vi "[FP] - VIG_Get Controls by Name.vi"(7 "MAin Ref\nFirst Time Only":refnum<vi>, 8 "Error":errorcluster, 11 "Control Names":string[](array[string])) -> (0 "Error Out":errorcluster, 3 "FP Controls Out":refnum<vi>[](array[refnum]), 5 "FrontPanel Out":refnum<vi>)   [LabVIEW 2015]
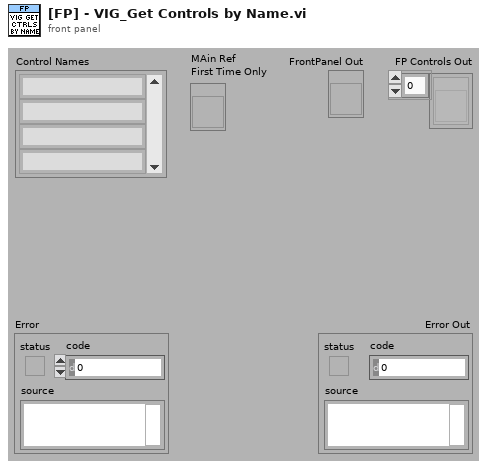
[diagram p1: front panel]
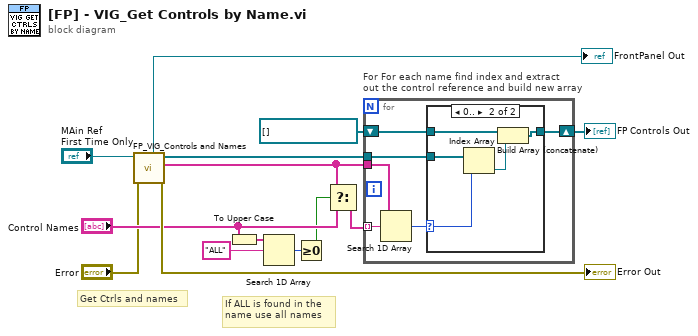
[diagram p0: block diagram]
diagram:
  # "If ALL is found in the\nname use all names"
  # "Get Ctrls and names"
  n1 = call "FP_VIG_Controls and Names.vi"("Error"="Error", "MAin Ref\nFirst Time only"="MAin Ref\nFirst Time Only") -> ("Error Out"=→"Error Out":errorcluster, "FP Names Out"=w8:string[], "FP Controls Out"=w3:refnum<vi>[], "FrontPanel Out"=→"FrontPanel Out":refnum<vi>)  [unwired: 6 in]
  n2 = To Upper Case(1:"Control Names") -> (0:w5:string[])
  n3 = Search 1D Array(1D array=w5, element="ALL") -> (index of element=w6:i32)  [unwired: 1 in]
  n4 = Greater Or Equal To 0?(x=w6) -> (x >= 0?=w7:bool)
  n5 = Select(t=w8, s=w7, f="Control Names") -> (s? t:f=w10:string[])
  n6 = for "For For each name find index and extract\nout the control reference and build new array" {
    tunnel: w8 -> [w20]
    tunnel: w10 -> [w19] mode=indexing
    tunnel: w3 -> [w17]
    shift-right: [w16] -> w14
    shift-left: refnum<vi>[] [] -> [w15]
    n7 = Search 1D Array(1D array=w20, element=w19) -> (index of element=w18:i32)  [unwired: 1 in]
    n8 = case shown="0.." w18 {
      selector: w18 -> [_ w25]
      tunnel: w17 -> [_ w26]
      tunnel: [w21 w23] -> w16
      tunnel: w15 -> [w21 w22]
      frame ..-1 {
      }
      frame 0.. {
        n9 = Index Array(array=w26, index=w25) -> (element=w24:refnum<vi>)
        n10 = Build Array (concatenate)(w22, w24) -> (w23:refnum<vi>[])
      }
    }
  }
  "FP Controls Out" <- w14
